vi "SeCrTs-DO_Write.vi"(7 "Data FIFO Ref":T1, 8 "error in (no error)":errorcluster, 11 "Refnum in":refnum<k21>) -> (0 "error out":errorcluster, 3 "Refnum out":refnum<k21>)   [LabVIEW 2022 SP3]
uses:
  RT Controls/SeCrTs-Data FIFO.ctl
  <vilib>/Platform/TimedLoop/XDataNode/timing_clust.ctl
  <vilib>/Platform/TimedLoop/XDataNode/nitl_modes.ctl
  <vilib>/Platform/TimedLoop/XDataNode/wakeup.ctl
  <vilib>/DAQmx/write.llb/DAQmx Write (Digital 1D Bool NChan 1Samp 1Line).vi
  <vilib>/DAQmx/miscellaneous.llb/DAQmx Fill In Error Info.vi
  <vilib>/platform/TimedLoop/XDataNode/XDataNode.xnode
  <vilib>/Platform/TimedLoop/XDataNode/XDNodeRunTimeDep.lvlib
panel:
  out "x":u32
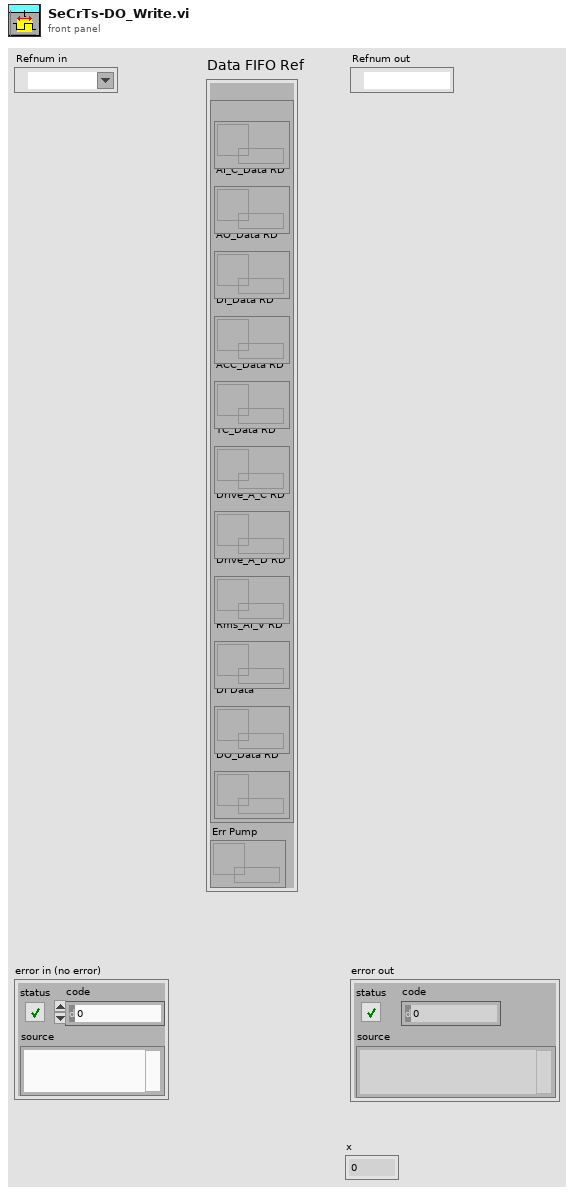
[diagram p1: front panel]
types:
  T1 = typedef "SeCrTs-Data FIFO.ctl" = cluster{"RD":cluster{"AI_V_Data RD":refnum<queue>, "AI_C_Data RD":refnum<queue>, "AO_Data RD":refnum<queue>, "DI_Data RD":refnum<queue>, "ACC_Data RD":refnum<queue>, "TC_Data RD":refnum<queue>, "Drive_A_C RD":refnum<queue>, "Drive_A_D RD":refnum<queue>, "Rms_AI_V RD":refnum<queue>, "DI Data":refnum<queue>, "DO_Data RD":refnum<queue>}, "Err Pump":refnum<queue>}
  T2 = typedef "XDNodeRunTimeDep.lvlib/timing_clust.ctl" = cluster{"Expected End [f-1]":u64, "Actual End [f-1]":u64, "Finished Late? [f-1]":bool, "Expected End [i-1]":u64, "Actual End [i-1]":u64, "Finished Late? [i-1]":bool, "Expected Start [i]":u64, "Actual Start [i]":u64, "Expected Start [f]":u64, "Actual Start [f]":u64, "Source Name":string, "Structure Name":string, "Period":i64, "Deadline":i64, "Offset":i64, "Start":i64, "Priority":i32, "Timeout":i32, "Mode":T3, "Wakeup Reason":T4, "Error":errorcluster, "Source Type":string, "Secondary Source Type":string, "Global End Time":u64, "Global Start Time":u64, "Frame Duration":u64, "Iteration Duration":u64, "Assigned CPU":i32, "I/O Scan Engine Mode":u32}
  T3 = typedef "XDNodeRunTimeDep.lvlib/nitl_modes.ctl" = enum32{"No Change", "Process missed periods, maintain original phase", "Discard missed periods, maintain original phase", "Process missed periods, ignore original phase", "Discard missed periods, ignore original phase"}
  T4 = typedef "XDNodeRunTimeDep.lvlib/wakeup.ctl" = enum32{"Normal", "Aborted", "Asynchronous wakeup", "Timing source error", "Timed loop error", "Timeout"}
  T5 = enum16{"AI C", "AI V", "AO", "DI", "DO", "TC", "ACC", "RT PMP", "DR A"}
  T6 = enum16{"Init", "Read", "Write 'All'", "Write 'n'", "Write Safe Value", "Write Start Time", "Overwrite Pattern", "Overwrite Pattern with Start", "Append Pattern", "Start Pattern Mode", "Abort Pattern Mode", "Read 1"}
  T7 = enum16{"Init", "Read 'All'", "Read 'n'", "Read '1'", "Write '1'", "Write 'n'", "Write 'All'"}
  T8 = cluster{"Start DAQ":bool, "Stop DAQ":bool, "RT Stop":bool, "RT Exit":bool, "Start Seq":bool}
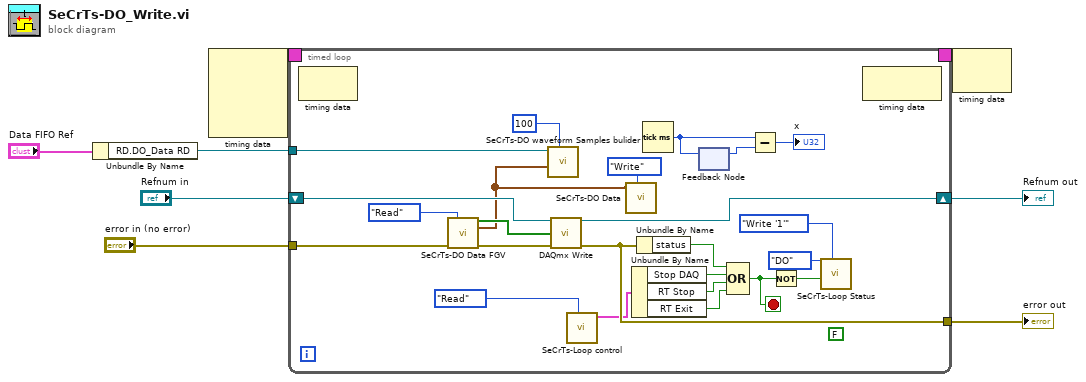
[diagram p0: block diagram]
diagram:
  n1 = Unbundle By Name("Data FIFO Ref") -> ("RD.DO_Data RD"=w3:refnum<queue>)
  n2 = node-c288() -> (w2:T2)  [unwired: 4 in]
  n3 = timed-loop {
    tunnel: "error in (no error)" -> [w21]
    tunnel: [w31] -> w7
    shift-right: [w19] -> w5
    shift-left: "Refnum in" -> [w30]
    tunnel: w3 -> [w14]
    timing: w2 -> [_]
    timing-out: [_] -> w1
    stop <- w32 stop-if-true
    (unwired) FALSE ("status")
    n4 = node-c288() -> ()  [unwired: 1 in, 1 out]
    n5 = call "SeCrTs-DO Data FGV.vi"("Option"=T6."Read", "error in (no error)"=w21) -> ("DO Values Out"=w18:bool[], "All data out"=w10:waveform(dbl)[], "error out"=w20:errorcluster)  [unwired: 7 in, 4 out]
    n6 = call "SeCrTs-DO waveform Samples bulider .vi"("Samples 2"=100 ("Samples"), "Data input 2"=w10, "DO_Data RD"=w14) -> ()  [unwired: 7 in, 2 out]
    n7 = call-poly <vilib>:"DAQmx Write.vi"("task/channels in"=w30, "data"=w18, "error in"=w20) -> ("task out"=w19:refnum<k21>, "error out"=w31:errorcluster)  [unwired: 10 in, 1 out]
    n8 = call "SeCrTs-Loop control.vi"("Action"=enum16{"Init", "Write", "Read"}."Read") -> ("Loop Control out"=w28:T8)  [unwired: 9 in, 1 out]
    n9 = call "SeCrTs-DO Data.vi"("Enum"=enum16{"Write", "Read"}."Write", "In_DO data"=w10) -> ()  [unwired: 9 in, 1 out]
    n10 = Unbundle By Name(w28) -> ("Stop DAQ"=w27:bool, "RT Stop"=w26:bool, "RT Exit"=w25:bool)
    n11 = Unbundle By Name(w31) -> ("status"=w29:bool)
    n12 = Tick Count (ms)() -> (millisecond timer value=w17:u32)
    n13 = feedback-in #1(w17) -> ()
    n14 = feedback #1() -> (w16:u32)  [unwired: 1 in]
    n15 = Compound Arithmetic op=OR(w29, w27, w26, w25) -> (w32:bool)
    n16 = Subtract(x=w17, y=w16) -> (x-y=→"x":u32)
    n17 = Not(x=w32) -> (.not. x?=w23:bool)
    n18 = call "SeCrTs-Loop Status.vi"("Option"=T7."Write '1'", "Status"=w23, "Loop"=T5."DO") -> ()  [unwired: 6 in, 3 out]
    n19 = node-c288() -> ()  [unwired: 1 in, 1 out]
  }
  "Refnum out" <- w5
  "error out" <- w7
  n20 = node-c288(w1) -> ()  [unwired: 1 out]
